vi "DSF.Engine.Execution.Transfer.RT FIFO.Read.vi"(8 "error in (no error)":errorcluster, 9 "timeout in ms (0)":i32, 11 "Transfer FIFO in":T1) -> (0 "error out":errorcluster, 1 "timed out?":bool, 2 "Transfer":refnum<class "DSF.Engine.Execution.Transfer.lvclass">, 3 "Transfer FIFO out":T1)   [LabVIEW 2016, in "DSF.Engine.lvlib" / "DSF.Engine.Execution.Transfer.lvclass"]
uses:
  DSF.Engine.Execution.Transfer.lvclass
  DSF.Engine.Execution.Transfer.RT FIFO Ref.ctl
  DSF.Engine.Execution.Transfer.RT FIFO Data.ctl
  DSF.Engine.Execution.Transfer.lvclass/DSF.Engine.Execution.Transfer.ctl
  Submodules/Memory/Source/Classes/Pointer/Memory.Pointer.lvclass/Memory.Pointer.ctl
  DSF.Engine.Execution.Transfer.Set Buffer.vi
  DSF.Engine.Execution.Transfer.Set ID.vi
  Buffer/DSF.Engine.Memory.Buffer.Block Descriptor.From.vi
  Submodules/Memory/Source/Classes/Pointer/Memory.Pointer.Block Descriptor to Object.vi
  Submodules/Memory/Source/Classes/Pointer/Memory.Pointer.Set Address.vi
  Submodules/Memory/Source/Classes/Pointer/Memory.Pointer.Set Size.vi
  Submodules/Memory/Source/Classes/Pointer/Memory.Pointer.Parameter Check.Null Pointer.vi
  Submodules/Memory/Source/Classes/Pointer/Memory.Pointer.Errors.vi
  Submodules/Memory/Source/Classes/Pointer/Memory.Pointer.Errors.Null Pointer.vi
  Submodules/Memory/Source/Classes/Pointer/Memory.Pointer.Get Address.vi
  Submodules/Memory/Source/Classes/Pointer/Memory.Pointer.Errors.Create Error.vi
  Submodules/Memory/Source/Submodules/SEH/Source/VIs/Static Error Handling.Error Cluster Constant.vi
  Submodules/Memory/Source/Submodules/SEH/Source/VIs/Static Error Handling.Error Cluster Constant (256B).vi
  Submodules/Memory/Source/Submodules/SEH/Source/VIs/Static Error Handling.Parameters.Status.Set.vi
  Submodules/Memory/Source/Submodules/SEH/Source/VIs/Static Error Handling.Parameters.Code.Set.vi
  Submodules/Memory/Source/Submodules/SEH/Source/VIs/Static Error Handling.Parameters.VI Source.Set.vi
  Submodules/Memory/Source/Constants/Memory.Constants.vi
  Submodules/Memory/Source/Constants/Memory.Constants.Library Name.vi
  Submodules/Memory/Source/Classes/Pointer/Memory.Pointer.Errors.Get Info.vi
  Submodules/Memory/Source/Submodules/SEH/Source/VIs/Static Error Handling.Source Buffer.Write.String.vi
  Buffer/DSF.Engine.Memory.Buffer.lvclass
  C:/Git/SourceTree/DSF/Source/Submodules/Memory/Source/Classes/Pointer/Memory.Pointer.lvclass
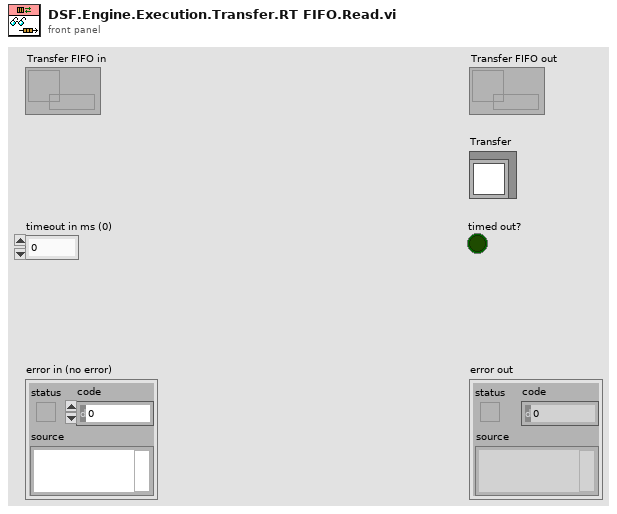
[diagram p1: front panel]
types:
  T1 = typedef "DSF.Engine.lvlib/DSF.Engine.Execution.Transfer.lvclass/DSF.Engine.Execution.Transfer.RT FIFO Ref.ctl" = refnum<k33>
  T2 = typedef "DSF.Engine.lvlib/DSF.Engine.Execution.Transfer.lvclass/DSF.Engine.Execution.Transfer.RT FIFO Data.ctl" = cluster{"ID":i32, "Buffer Descriptor":cluster{"address":u64, "size":u64}}
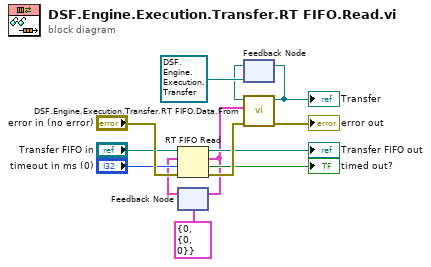
[diagram p0: block diagram]
diagram:
  n1 = feedback #1(T2 {"ID"=0, "Buffer Descriptor"={"address"=0, "size"=0}} ("element")) -> (w4:T2)
  n2 = RT FIFO Read(0:"Transfer FIFO in", 1:w4, 2:"timeout in ms (0)", 3:"error in (no error)") -> (8:→"Transfer FIFO out":T1, 9:w2:T2, 10:→"timed out?":bool, 11:w8:errorcluster)  [unwired: 1 out]
  n3 = feedback-in #1(w2) -> ()
  n4 = feedback #2(refnum<class "DSF.Engine.Execution.Transfer.lvclass"> refnum ("Transfer out")) -> (w1:refnum<class "DSF.Engine.Execution.Transfer.lvclass">)
  n5 = call "DSF.Engine.Execution.Transfer.RT FIFO.Data.From.vi"("error in (no error)"=w8, "Transfer Data"=w2, "Transfer in"=w1) -> ("error out"=→"error out":errorcluster, "Transfer out"=w6:refnum<class "DSF.Engine.Execution.Transfer.lvclass">)  [unwired: 7 in]
  "Transfer" <- w6
  n6 = feedback-in #2(w6) -> ()
